vi "S4GUI_003.vi"(7 "Tab ObsEng":enum32{"Obs", "CCD modes", "Guider", "Eng"}(tab)) -> ()   [LabVIEW 2018] (continued)
                    n552 = To Long Integer(number=w1145) -> (32bit integer=w1147:i32)
                    n553 = Subtract(x=w1147, y=w1146) -> (x-y=w1148:i32)
                    n554 = Decrement(x=w1148) -> (x-1=w1150:i32)
                    n555 = Less Than 0?(x=w1150) -> (x < 0?=w1149:bool)
                    n556 = Select(t=0, s=w1149, f=w1150) -> (s? t:f=w1151:i32)
                  }
                }
                "#Pol. Seq. Done" <- w1134
                n557 = Number To Decimal String(number=w1134) -> (decimal integer string=w1135:string)  [unwired: 1 in]
                n558 = Concatenate Strings("#Pol. Seq. Done ", w1135) -> (w1133:string)
                n559 = property on="#Pol. Seq. Done" class="Slide (strict)"("Caption.Text"=w1133) -> ()  [unwired: 2 in, 2 out]
              }
              frame #10 {
                # "OVJ 2022-12-12: \nA visibilidade do Tab ObsEng sempre \nacompanha a habilitação do tab4."
                n560 = Unbundle By Name(w1165) -> ("Cluster ExpMode.tab4"=w1159:T12, "Cluster Polarimetry"=w1186:T23, "Cluster Mode Sync"=w1193:T24)
                n561 = case shown="\"Enabled\", Default" w1159 {
                  tunnel: [TRUE ("Tabs Visible?") w1195] -> w1164
                  frame "Enabled", Default {
                  }
                  frame "Disabled and Grayed Out" {
                    n562 = disable-structure shown="Enabled" {
                      disable-tunnel: [TRUE ("Tabs Visible?") FALSE ("Tabs Visible?")] -> w1195
                      frame Disabled {
                        # "DEBUG"
                      }
                      frame Enabled {
                      }
                    }
                  }
                }
                n563 = property on="Tab Acq Type" class="TabCtl (strict)"("DisabledEnum"=w1159) -> (error out=w1163:errorcluster)  [unwired: 2 in, 1 out]
                n564 = Unbundle By Name(w1193) -> ("Start SM Text"=w1192:string, "Star SM"=w1161:T12, "Pause SM"=w1191:T12, "Stop SM"=w1190:T12, "Abort SM"=w1189:T12, "#Cycles"=w1188:T12, "SSM"=w1187:T12, "Set SM"=w1156:T12, "#Index Cycles"=w1162:T12)
                n565 = property on="Observer" class="Str"(error in=w1163, "DisabledEnum"=w1159) -> (error out=w1158:errorcluster)  [unwired: 1 in, 1 out]
                n566 = property on="Tab ObsEng" class="TabCtl (strict)"("Tabs Visible?"=w1164) -> ()  [unwired: 2 in, 2 out]
                n567 = property on="Project ID" class="Str"(error in=w1158, "DisabledEnum"=w1159) -> (error out=w1157:errorcluster)  [unwired: 1 in, 1 out]
                n568 = property on="set keywords" class="Bool"(error in=w1157, "DisabledEnum"=w1156) -> (error out=w1160:errorcluster)  [unwired: 1 in, 1 out]
                n569 = property on="Start SM" class="Bool"("BoolText.Text"=w1192) -> ()  [unwired: 2 in, 2 out]
                n570 = property on="#Cycles Done" class="Slide (strict)"("DisabledEnum"=w1162) -> ()  [unwired: 2 in, 2 out]
                n571 = property on="Start SM" class="Bool"("DisabledEnum"=w1161) -> ()  [unwired: 2 in, 2 out]
                n572 = property on="Stop SM" class="Bool"("DisabledEnum"=w1190) -> ()  [unwired: 2 in, 2 out]
                n573 = property on="Abort SM" class="Bool"("DisabledEnum"=w1189) -> ()  [unwired: 2 in, 2 out]
                n574 = property on="Pause SM" class="Bool"("DisabledEnum"=w1191) -> ()  [unwired: 2 in, 2 out]
                n575 = property on="# Cycles" class="DigNum (strict)"("DisabledEnum"=w1188) -> ()  [unwired: 2 in, 2 out]
                n576 = property on="SSM" class="Ring (strict)"("DisabledEnum"=w1187) -> ()  [unwired: 2 in, 2 out]
                n577 = property on="set Observer" class="Bool"(error in=w1160, "DisabledEnum"=w1156) -> ()  [unwired: 1 in, 2 out]
                n578 = Unbundle By Name(w1186) -> ("Lambda Selector"=w1185:T12, "Calibrator Selector"=w1184:T12, "Set Waveplate"=w1183:T12, "Select Positions"=w1182:T12, "P0"=w1181:T12, "P8"=w1180:T12, "P1"=w1179:T12, "P9"=w1178:T12, "P2"=w1177:T12, "P10"=w1176:T12, "P3"=w1175:T12, "P11"=w1174:T12, "P4"=w1173:T12, "P12"=w1172:T12, "P5"=w1171:T12, "P13"=w1170:T12, "P6"=w1169:T12, "P14"=w1168:T12, "P7"=w1167:T12, "P15"=w1166:T12)
                n579 = property on="P0" class="Bool (strict)"("DisabledEnum"=w1181) -> ()  [unwired: 2 in, 2 out]
                n580 = property on="Lambda Selector" class="Ring (strict)"("DisabledEnum"=w1185) -> ()  [unwired: 2 in, 2 out]
                n581 = property on="Calibrator Selector" class="Ring (strict)"("DisabledEnum"=w1184) -> ()  [unwired: 2 in, 2 out]
                n582 = property on="Set Waveplate" class="Bool"("DisabledEnum"=w1183) -> ()  [unwired: 2 in, 2 out]
                n583 = property on="P1" class="Bool (strict)"("DisabledEnum"=w1179) -> ()  [unwired: 2 in, 2 out]
                n584 = property on="P2" class="Bool (strict)"("DisabledEnum"=w1177) -> ()  [unwired: 2 in, 2 out]
                n585 = property on="Select Positions" class="Ring (strict)"("DisabledEnum"=w1182) -> ()  [unwired: 2 in, 2 out]
                n586 = property on="P3" class="Bool (strict)"("DisabledEnum"=w1175) -> ()  [unwired: 2 in, 2 out]
                n587 = property on="P4" class="Bool (strict)"("DisabledEnum"=w1173) -> ()  [unwired: 2 in, 2 out]
                n588 = property on="P5" class="Bool (strict)"("DisabledEnum"=w1171) -> ()  [unwired: 2 in, 2 out]
                n589 = property on="P6" class="Bool (strict)"("DisabledEnum"=w1169) -> ()  [unwired: 2 in, 2 out]
                n590 = property on="P7" class="Bool (strict)"("DisabledEnum"=w1167) -> ()  [unwired: 2 in, 2 out]
                n591 = property on="P8" class="Bool (strict)"("DisabledEnum"=w1180) -> ()  [unwired: 2 in, 2 out]
                n592 = property on="P9" class="Bool (strict)"("DisabledEnum"=w1178) -> ()  [unwired: 2 in, 2 out]
                n593 = property on="P10" class="Bool (strict)"("DisabledEnum"=w1176) -> ()  [unwired: 2 in, 2 out]
                n594 = property on="P11" class="Bool (strict)"("DisabledEnum"=w1174) -> ()  [unwired: 2 in, 2 out]
                n595 = property on="P12" class="Bool (strict)"("DisabledEnum"=w1172) -> ()  [unwired: 2 in, 2 out]
                n596 = property on="P15" class="Bool (strict)"("DisabledEnum"=w1166) -> ()  [unwired: 2 in, 2 out]
                n597 = property on="P13" class="Bool (strict)"("DisabledEnum"=w1170) -> ()  [unwired: 2 in, 2 out]
                n598 = property on="P14" class="Bool (strict)"("DisabledEnum"=w1168) -> ()  [unwired: 2 in, 2 out]
              }
              frame #11 {
                n599 = Unbundle By Name(w1212) -> ("Cluster Mode CH1"=w1200:T25, "Cluster Mode Sync"=w1199:T24)
                n600 = Unbundle By Name(w1200) -> ("Start ch1 Text"=w1211:string, "#cycles ch1"=w1210:T12, "Start ch1"=w1209:T12, "Pause ch1"=w1208:T12, "Abort ch1"=w1207:T12, "Stop ch1"=w1206:T12, "Exptime ch1"=w1205:T12, "Exp ch1"=w1204:T12, "Set Cooler"=w1198:T12, "Set Temp"=w1203:T12)
                n601 = Unbundle By Name(w1199) -> ("#Index Cycles"=w1202:T12)
                n602 = case shown="Default" w1202 {
                  tunnel: [T12."Enabled" ("#Index Cycles") T12."Disabled and Grayed Out" ("#Index Cycles")] -> w1201
                  frame "Disabled and Grayed Out" {
                  }
                  frame Default {
                  }
                }
                n603 = property on="Start ch1" class="Bool"("BoolText.Text"=w1211) -> ()  [unwired: 2 in, 2 out]
                n604 = property on="Abort ch1" class="Bool"("DisabledEnum"=w1207) -> ()  [unwired: 2 in, 2 out]
                n605 = property on="Set Temp 1" class="Bool"("DisabledEnum"=w1203) -> ()  [unwired: 2 in, 2 out]
                n606 = property on="Stop ch1" class="Bool"("DisabledEnum"=w1206) -> ()  [unwired: 2 in, 2 out]
                n607 = property on="#cycles ch1" class="DigNum (strict)"("DisabledEnum"=w1210) -> ()  [unwired: 2 in, 2 out]
                n608 = property on="cooler ON 1" class="Bool (strict)"("DisabledEnum"=w1198) -> ()  [unwired: 2 in, 2 out]
                n609 = property on="cooler OFF 1" class="Bool (strict)"("DisabledEnum"=w1198) -> ()  [unwired: 2 in, 2 out]
                n610 = property on="Exptime ch1" class="DigNum (strict)"("DisabledEnum"=w1205) -> ()  [unwired: 2 in, 2 out]
                n611 = property on="Start ch1" class="Bool"("DisabledEnum"=w1209) -> ()  [unwired: 2 in, 2 out]
                n612 = property on="Exp ch1" class="DigNum (strict)"("DisabledEnum"=w1204) -> ()  [unwired: 2 in, 2 out]
                n613 = property on="Cycles Done ch1" class="Slide (strict)"("DisabledEnum"=w1201) -> ()  [unwired: 2 in, 2 out]
                n614 = property on="Pause ch1" class="Bool"("DisabledEnum"=w1208) -> ()  [unwired: 2 in, 2 out]
              }
              frame #12 {
                n615 = Unbundle By Name(w1229) -> ("Cluster Mode CH2"=w1228:T26, "Cluster Mode Sync"=w1217:T24)
                n616 = Unbundle By Name(w1217) -> ("#Index Cycles"=w1218:T12)
                n617 = Unbundle By Name(w1228) -> ("Start ch2 Text"=w1227:string, "#cycles ch2"=w1226:T12, "Start ch2"=w1225:T12, "Pause ch2"=w1224:T12, "Stop ch2"=w1223:T12, "Abort ch2"=w1222:T12, "Exptime ch2"=w1221:T12, "Exp ch2"=w1220:T12, "Set Cooler"=w1215:T12, "Set Temp"=w1219:T12)
                n618 = case shown="\"Disabled and Grayed Out\"" w1218 {
                  tunnel: [T12."Enabled" ("#Index Cycles") T12."Disabled and Grayed Out" ("#Index Cycles")] -> w1216
                  frame "Disabled and Grayed Out" {
                  }
                  frame Default {
                  }
                }
                n619 = property on="Start ch2" class="Bool"("BoolText.Text"=w1227) -> ()  [unwired: 2 in, 2 out]
                n620 = property on="Stop ch2" class="Bool"("DisabledEnum"=w1223) -> ()  [unwired: 2 in, 2 out]
                n621 = property on="Abort ch2" class="Bool"("DisabledEnum"=w1222) -> ()  [unwired: 2 in, 2 out]
                n622 = property on="#cycles ch2" class="DigNum (strict)"("DisabledEnum"=w1226) -> ()  [unwired: 2 in, 2 out]
                n623 = property on="Set Temp 2" class="Bool"("DisabledEnum"=w1219) -> ()  [unwired: 2 in, 2 out]
                n624 = property on="Exptime ch2" class="DigNum (strict)"("DisabledEnum"=w1221) -> ()  [unwired: 2 in, 2 out]
                n625 = property on="cooler OFF 2" class="Bool (strict)"("DisabledEnum"=w1215) -> ()  [unwired: 2 in, 2 out]
                n626 = property on="cooler ON 2" class="Bool (strict)"("DisabledEnum"=w1215) -> ()  [unwired: 2 in, 2 out]
                n627 = property on="Start ch2" class="Bool"("DisabledEnum"=w1225) -> ()  [unwired: 2 in, 2 out]
                n628 = property on="Cycles Done ch2" class="Slide (strict)"("DisabledEnum"=w1216) -> ()  [unwired: 2 in, 2 out]
                n629 = property on="Exp ch2" class="DigNum (strict)"("DisabledEnum"=w1220) -> ()  [unwired: 2 in, 2 out]
                n630 = property on="Pause ch2" class="Bool"("DisabledEnum"=w1224) -> ()  [unwired: 2 in, 2 out]
              }
              frame #13 {
                n631 = Unbundle By Name(w1246) -> ("Cluster Mode CH3"=w1245:T27, "Cluster Mode Sync"=w1234:T24)
                n632 = Unbundle By Name(w1234) -> ("#Index Cycles"=w1235:T12)
                n633 = Unbundle By Name(w1245) -> ("Start ch3 Text"=w1244:string, "#cycles ch3"=w1243:T12, "Start ch3"=w1242:T12, "Pause ch3"=w1241:T12, "Stop ch3"=w1240:T12, "Abort ch3"=w1239:T12, "Exptime ch3"=w1238:T12, "Exp ch3"=w1237:T12, "Set Cooler"=w1232:T12, "Set Temp"=w1236:T12)
                n634 = case shown="\"Disabled and Grayed Out\"" w1235 {
                  tunnel: [T12."Enabled" ("#Index Cycles") T12."Disabled and Grayed Out" ("#Index Cycles")] -> w1233
                  frame "Disabled and Grayed Out" {
                  }
                  frame Default {
                  }
                }
                n635 = property on="Start ch3" class="Bool"("BoolText.Text"=w1244) -> ()  [unwired: 2 in, 2 out]
                n636 = property on="Stop ch3" class="Bool"("DisabledEnum"=w1240) -> ()  [unwired: 2 in, 2 out]
                n637 = property on="Abort ch3" class="Bool"("DisabledEnum"=w1239) -> ()  [unwired: 2 in, 2 out]
                n638 = property on="Cycles Done ch3" class="Slide (strict)"("DisabledEnum"=w1233) -> ()  [unwired: 2 in, 2 out]
                n639 = property on="#cycles ch3" class="DigNum (strict)"("DisabledEnum"=w1243) -> ()  [unwired: 2 in, 2 out]
                n640 = property on="cooler OFF 3" class="Bool (strict)"("DisabledEnum"=w1232) -> ()  [unwired: 2 in, 2 out]
                n641 = property on="Set Temp 3" class="Bool"("DisabledEnum"=w1236) -> ()  [unwired: 2 in, 2 out]
                n642 = property on="cooler ON 3" class="Bool (strict)"("DisabledEnum"=w1232) -> ()  [unwired: 2 in, 2 out]
                n643 = property on="Exptime ch3" class="DigNum (strict)"("DisabledEnum"=w1238) -> ()  [unwired: 2 in, 2 out]
                n644 = property on="Start ch3" class="Bool"("DisabledEnum"=w1242) -> ()  [unwired: 2 in, 2 out]
                n645 = property on="Exp ch3" class="DigNum (strict)"("DisabledEnum"=w1237) -> ()  [unwired: 2 in, 2 out]
                n646 = property on="Pause ch3" class="Bool"("DisabledEnum"=w1241) -> ()  [unwired: 2 in, 2 out]
              }
              frame #14 {
                n647 = Unbundle By Name(w1263) -> ("Cluster Mode CH4"=w1262:T28, "Cluster Mode Sync"=w1251:T24)
                n648 = Unbundle By Name(w1251) -> ("#Index Cycles"=w1252:T12)
                n649 = Unbundle By Name(w1262) -> ("Start ch4 Text"=w1261:string, "#cycles ch4"=w1260:T12, "Start ch4"=w1259:T12, "Pause ch4"=w1258:T12, "Stop ch4"=w1257:T12, "Abort ch4"=w1256:T12, "Exptime ch4"=w1255:T12, "Exp ch4"=w1254:T12, "Set Cooler"=w1249:T12, "Set Temp"=w1253:T12)
                n650 = case shown="\"Disabled and Grayed Out\"" w1252 {
                  tunnel: [T12."Enabled" ("#Index Cycles") T12."Disabled and Grayed Out" ("#Index Cycles")] -> w1250
                  frame "Disabled and Grayed Out" {
                  }
                  frame Default {
                  }
                }
                n651 = property on="Start ch4" class="Bool"("BoolText.Text"=w1261) -> ()  [unwired: 2 in, 2 out]
                n652 = property on="Stop ch4" class="Bool"("DisabledEnum"=w1257) -> ()  [unwired: 2 in, 2 out]
                n653 = property on="Abort ch4" class="Bool"("DisabledEnum"=w1256) -> ()  [unwired: 2 in, 2 out]
                n654 = property on="#cycles ch4" class="DigNum (strict)"("DisabledEnum"=w1260) -> ()  [unwired: 2 in, 2 out]
                n655 = property on="Set Temp 4" class="Bool"("DisabledEnum"=w1253) -> ()  [unwired: 2 in, 2 out]
                n656 = property on="cooler ON 4" class="Bool (strict)"("DisabledEnum"=w1249) -> ()  [unwired: 2 in, 2 out]
                n657 = property on="cooler OFF 4" class="Bool (strict)"("DisabledEnum"=w1249) -> ()  [unwired: 2 in, 2 out]
                n658 = property on="Exptime ch4" class="DigNum (strict)"("DisabledEnum"=w1255) -> ()  [unwired: 2 in, 2 out]
                n659 = property on="Cycles Done ch4" class="Slide (strict)"("DisabledEnum"=w1250) -> ()  [unwired: 2 in, 2 out]
                n660 = property on="Start ch4" class="Bool"("DisabledEnum"=w1259) -> ()  [unwired: 2 in, 2 out]
                n661 = property on="Exp ch4" class="DigNum (strict)"("DisabledEnum"=w1254) -> ()  [unwired: 2 in, 2 out]
                n662 = property on="Pause ch4" class="Bool"("DisabledEnum"=w1258) -> ()  [unwired: 2 in, 2 out]
              }
              frame #15 {
                # "Carrega coluna do Channel 1"
                # "Aba:  Eng->Camera"
                n663 = Unbundle By Name(w1330) -> ("ChannelA_CCD"=w1275:T29, "CHA_Checked Params"=w1321:T14, "ChannelA_Status.connection"=w1274:bool)
                n664 = Unbundle By Name(w1321) -> ("ACQUISITION_MODE"=w1299:bool, "TRIGGER_MODE"=w1300:bool, "READ_MODE"=w1301:bool, "PREAMP"=w1309:bool, "READOUT_RATE"=w1310:bool, "VERTICAL_SHIFT_SPEED"=w1311:bool, "EM_MODE"=w1312:bool, "EM_GAIN"=w1302:bool, "SHUTTER_MODE"=w1303:bool, "SHUTTER_TTL"=w1304:bool, "SHUTTER_OPENING_TIME"=w1305:bool, "SHUTTER_CLOSING_TIME"=w1306:bool, "VBIN"=w1307:bool, "HBIN"=w1308:bool, "INITIAL_LINE"=w1313:bool, "INITIAL_COLUMN"=w1318:bool, "FINAL_LINE"=w1320:bool, "FINAL_COLUMN"=w1317:bool, "FRAME_TRANSFER"=w1316:bool, "VERTICAL_CLOCK_VOLTAGE"=w1315:bool, "AD_CHANNEL"=w1314:bool)
                n665 = local read "CH1on"() -> (w1267:bool)
                n666 = Unbundle By Name(w1275) -> ("INITIAL_LINE"=w1297:u16, "INITIAL_COLUMN"=w1296:u16, "FINAL_LINE"=w1295:u16, "FINAL_COLUMN"=w1294:u16, "VBIN"=w1293:u16, "HBIN"=w1292:u16, "PREAMP"=w1291:u8, "EM_GAIN"=w1290:u16, "READOUT_RATE"=w1289:u8, "SHUTTER_OPENNING_TIME"=w1288:u16, "SHUTTER_CLOSING_TIME"=w1287:u16, "VERTICAL_SHIFT_SPEED"=w1286:u8, "READ_MODE"=w1285:u8, "VERTICAL_CLOCK_VOLTAGE"=w1284:u8, "AD_CHANNEL"=w1283:u32, "SHUTTER_MODE"=w1282:u8, "SHUTTER_TTL"=w1281:u8, "TRIGGER_MODE"=w1280:u8, "FRAME_TRANSFER"=w1279:bool, "ACQUISITION_MODE"=w1277:u8, "EM_MODE"=w1276:u8)
                n667 = Equal?(x=w1325, y="none") -> (x = y?=w1322:bool)
                n668 = Equal?(x=w1325, y="default.cfg") -> (x = y?=w1323:bool)
                n669 = Or(x=w1323, y=w1322) -> (x .or. y?=w1324:bool)
                n670 = case shown="True" w1324 {
                  tunnel: [T12."Enabled" ("Disabled") T12."Disabled and Grayed Out" ("Disabled")] -> w1327
                  frame False {
                    # "Se Curr Conf File != default.cfg,\nhabilita botão de Salvar."
                  }
                  frame True {
                    # "Não é permitido salvar em \ncima de default.cfg"
                  }
                }
                n671 = case shown="True" w1274 {
                  tunnel: w1275 -> [_ w1383]
                  tunnel: [w1376 w1382] -> w1273
                  tunnel: [w1376 w1381] -> w1272
                  tunnel: [w1376 w1380] -> w1271
                  tunnel: [w1376 w1379] -> w1270
                  tunnel: [w1376 w1378] -> w1269
                  tunnel: [w1376 w1377] -> w1268
                  frame False {
                    w1376 = "" ("RO1")
                  }
                  frame True {
                    n672 = stacked-sequence "Atualizacao dos indicadores inferiores do CANAL A da tela principal" {
                      tunnel: w1383 -> [w1398 w1401 w1406 w1415 w1418 w1422]
                      tunnel: [w1384 _ _ _ _ _] -> w1382
                      tunnel: [_ w1399 _ _ _ _] -> w1381
                      tunnel: [_ _ w1404 _ _ _] -> w1380
                      tunnel: [_ _ _ w1409 _ _] -> w1379
                      tunnel: [_ _ _ _ w1416 _] -> w1378
                      tunnel: [_ _ _ _ _ w1419] -> w1377
                      frame #0 {
                        # "SubImage"
                        n673 = Unbundle By Name(w1398) -> ("INITIAL_LINE"=w1396:u16, "FINAL_LINE"=w1395:u16, "INITIAL_COLUMN"=w1394:u16, "FINAL_COLUMN"=w1393:u16)
                        n674 = Number To Decimal String(number=w1396) -> (decimal integer string=w1392:string)  [unwired: 1 in]
                        n675 = Number To Decimal String(number=w1395) -> (decimal integer string=w1390:string)  [unwired: 1 in]
                        n676 = Number To Decimal String(number=w1394) -> (decimal integer string=w1388:string)  [unwired: 1 in]
                        n677 = Number To Decimal String(number=w1393) -> (decimal integer string=w1386:string)  [unwired: 1 in]
                        n678 = Concatenate Strings("[", w1392, ":", w1390, ",", w1388, ":", w1386, "]") -> (w1384:string)
                      }
                      frame #1 {
                        # "Em Active"
                        n679 = Unbundle By Name(w1401) -> ("EM_MODE"=w1400:u8)
                        n680 = case shown="0, Default" w1400 {
                          tunnel: ["Electron M." ("EmActive1") "Convent." ("EmActive1")] -> w1399
                          frame 0, Default {
                          }
                          frame 1 {
                          }
                        }
                      }
                      frame #2 {
                        # "Pre Amp"
                        n681 = Unbundle By Name(w1406) -> ("PREAMP"=w1405:u8)
                        n682 = case shown="1" w1405 {
                          tunnel: ["Gain 1" ("EmActive1") "Gain 2" ("EmActive1")] -> w1404
                          frame 0, Default {
                          }
                          frame 1 {
                          }
                        }
                      }
                      frame #3 {
                        # "Binning"
                        n683 = Unbundle By Name(w1415) -> ("VBIN"=w1414:u16, "HBIN"=w1413:u16)
                        n684 = Number To Decimal String(number=w1413) -> (decimal integer string=w1410:string)  [unwired: 1 in]
                        n685 = Number To Decimal String(number=w1414) -> (decimal integer string=w1412:string)  [unwired: 1 in]
                        n686 = Concatenate Strings(w1412, "x", w1410) -> (w1409:string)
                      }
                      frame #4 {
                        # "Gain"
                        n687 = Unbundle By Name(w1418) -> ("EM_GAIN"=w1417:u16)
                        n688 = Number To Decimal String(number=w1417) -> (decimal integer string=w1416:string)  [unwired: 1 in]
                      }
                      frame #5 {
                        # "Readout"
                        n689 = Unbundle By Name(w1422) -> ("EM_MODE"=w1421:u8, "READOUT_RATE"=w1420:u8)
                        n690 = case shown="0, Default" w1421 {
                          tunnel: w1420 -> [w1424 w1430]
                          tunnel: [w1423 w1429] -> w1419
                          frame 0, Default {
                            n691 = case shown="0, Default" w1424 {
                              tunnel: ["30 MHz" ("EmActive1") "20 MHz" ("EmActive1") "10 MHz" ("EmActive1") "1 MHz" ("EmActive1")] -> w1423
                              frame 0, Default {
                              }
                              frame 1 {
                              }
                              frame 2 {
                              }
                              frame 3 {
                              }
                            }
                          }
                          frame 1 {
                            n692 = case shown="1" w1430 {
                              tunnel: ["1 MHz" ("EmActive1") "0.1 MHz" ("EmActive1")] -> w1429
                              frame 0, Default {
                              }
                              frame 1 {
                              }
                            }
                          }
                        }
                      }
                    }
                  }
                }
                n693 = case shown="False" w1267 {
                  tunnel: w1320 -> [_ w1375]
                  tunnel: w1318 -> [_ w1371]
                  tunnel: w1317 -> [_ w1369]
                  tunnel: w1316 -> [_ w1365]
                  tunnel: w1315 -> [_ w1364]
                  tunnel: w1314 -> [_ w1363]
                  tunnel: w1313 -> [_ w1355]
                  tunnel: w1312 -> [_ w1347]
                  tunnel: w1311 -> [_ w1346]
                  tunnel: w1310 -> [_ w1345]
                  tunnel: w1309 -> [_ w1344]
                  tunnel: w1308 -> [_ w1343]
                  tunnel: w1307 -> [_ w1342]
                  tunnel: w1306 -> [_ w1341]
                  tunnel: w1305 -> [_ w1340]
                  tunnel: w1304 -> [_ w1339]
                  tunnel: w1303 -> [_ w1338]
                  tunnel: w1302 -> [_ w1337]
                  tunnel: w1301 -> [_ w1336]
                  tunnel: w1300 -> [_ w1335]
                  tunnel: w1299 -> [_ w1334]
                  tunnel: [T12."Disabled and Grayed Out" ("Disabled") T12."Enabled" ("Disabled")] -> w1266
                  frame False {
                    w1331 = FALSE
                    n694 = property on="Image FInal Column" class="DigNum (strict)"("Blinking"=w1331) -> ()  [unwired: 2 in, 2 out]
                    n695 = property on="Frame Transfer" class="Bool (strict)"("Blinking"=w1331) -> ()  [unwired: 2 in, 2 out]
                    n696 = property on="Vertical Clock Voltage" class="Ring (strict)"("Blinking"=w1331) -> ()  [unwired: 2 in, 2 out]
                    n697 = property on="A/D  Channel" class="DigNum (strict)"("Blinking"=w1331) -> ()  [unwired: 2 in, 2 out]
                    n698 = property on="Image Initial Line" class="DigNum (strict)"("Blinking"=w1331) -> ()  [unwired: 2 in, 2 out]
                    n699 = property on="Image Initial Column" class="DigNum (strict)"("Blinking"=w1331) -> ()  [unwired: 2 in, 2 out]
                    n700 = property on="Image Final Line" class="DigNum (strict)"("Blinking"=w1331) -> ()  [unwired: 2 in, 2 out]
                    n701 = property on="Shutter Openning Time" class="DigNum (strict)"("Blinking"=w1331) -> ()  [unwired: 2 in, 2 out]
                    n702 = property on="Shutter Closing Time" class="DigNum (strict)"("Blinking"=w1331) -> ()  [unwired: 2 in, 2 out]
                    n703 = property on="Vertical Binning" class="DigNum (strict)"("Blinking"=w1331) -> ()  [unwired: 2 in, 2 out]
                    n704 = property on="Horizontal Binning" class="DigNum (strict)"("Blinking"=w1331) -> ()  [unwired: 2 in, 2 out]
                    n705 = property on="CCD EM Gain" class="DigNum (strict)"("Blinking"=w1331) -> ()  [unwired: 2 in, 2 out]
                    n706 = property on="Shutter Mode" class="Ring (strict)"("Blinking"=w1331) -> ()  [unwired: 2 in, 2 out]
                    n707 = property on="Shutter TTL" class="Ring (strict)"("Blinking"=w1331) -> ()  [unwired: 2 in, 2 out]
                    n708 = property on="Acquisition Mode" class="Ring (strict)"("Blinking"=w1331) -> ()  [unwired: 2 in, 2 out]
                    n709 = property on="Readout Rate" class="Ring (strict)"("Blinking"=w1331) -> ()  [unwired: 2 in, 2 out]
                    n710 = property on="Vertical Shift Speed" class="Ring (strict)"("Blinking"=w1331) -> ()  [unwired: 2 in, 2 out]
                    n711 = property on="CCD EM Mode" class="Ring (strict)"("Blinking"=w1331) -> ()  [unwired: 2 in, 2 out]
                    n712 = property on="Trigger Mode" class="Ring (strict)"("Blinking"=w1331) -> ()  [unwired: 2 in, 2 out]
                    n713 = property on="Read Mode" class="Ring (strict)"("Blinking"=w1331) -> ()  [unwired: 2 in, 2 out]
                    n714 = property on="Pre-amplification Gain" class="Ring (strict)"("Blinking"=w1331) -> ()  [unwired: 2 in, 2 out]
                  }
                  frame True {
                    n715 = Not(x=w1369) -> (.not. x?=w1370:bool)
                    n716 = Not(x=w1365) -> (.not. x?=w1367:bool)
                    n717 = Not(x=w1364) -> (.not. x?=w1368:bool)
                    n718 = Not(x=w1363) -> (.not. x?=w1366:bool)
                    n719 = Not(x=w1355) -> (.not. x?=w1373:bool)
                    n720 = Not(x=w1371) -> (.not. x?=w1372:bool)
                    n721 = Not(x=w1375) -> (.not. x?=w1374:bool)
                    n722 = property on="Image FInal Column" class="DigNum (strict)"("Blinking"=w1370) -> ()  [unwired: 2 in, 2 out]
                    n723 = property on="Frame Transfer" class="Bool (strict)"("Blinking"=w1367) -> ()  [unwired: 2 in, 2 out]
                    n724 = property on="Vertical Clock Voltage" class="Ring (strict)"("Blinking"=w1368) -> ()  [unwired: 2 in, 2 out]
                    n725 = property on="A/D  Channel" class="DigNum (strict)"("Blinking"=w1366) -> ()  [unwired: 2 in, 2 out]
                    n726 = property on="Image Initial Line" class="DigNum (strict)"("Blinking"=w1373) -> ()  [unwired: 2 in, 2 out]
                    n727 = property on="Image Initial Column" class="DigNum (strict)"("Blinking"=w1372) -> ()  [unwired: 2 in, 2 out]
                    n728 = property on="Image Final Line" class="DigNum (strict)"("Blinking"=w1374) -> ()  [unwired: 2 in, 2 out]
                    n729 = Not(x=w1340) -> (.not. x?=w1359:bool)
                    n730 = Not(x=w1341) -> (.not. x?=w1361:bool)
                    n731 = Not(x=w1342) -> (.not. x?=w1360:bool)
                    n732 = Not(x=w1343) -> (.not. x?=w1362:bool)
                    n733 = Not(x=w1337) -> (.not. x?=w1357:bool)
                    n734 = Not(x=w1338) -> (.not. x?=w1358:bool)
                    n735 = Not(x=w1339) -> (.not. x?=w1356:bool)
                    n736 = property on="Shutter Openning Time" class="DigNum (strict)"("Blinking"=w1359) -> ()  [unwired: 2 in, 2 out]
                    n737 = property on="Shutter Closing Time" class="DigNum (strict)"("Blinking"=w1361) -> ()  [unwired: 2 in, 2 out]
                    n738 = property on="Vertical Binning" class="DigNum (strict)"("Blinking"=w1360) -> ()  [unwired: 2 in, 2 out]
                    n739 = property on="Horizontal Binning" class="DigNum (strict)"("Blinking"=w1362) -> ()  [unwired: 2 in, 2 out]
                    n740 = property on="CCD EM Gain" class="DigNum (strict)"("Blinking"=w1357) -> ()  [unwired: 2 in, 2 out]
                    n741 = property on="Shutter Mode" class="Ring (strict)"("Blinking"=w1358) -> ()  [unwired: 2 in, 2 out]
                    n742 = property on="Shutter TTL" class="Ring (strict)"("Blinking"=w1356) -> ()  [unwired: 2 in, 2 out]
                    n743 = Not(x=w1334) -> (.not. x?=w1348:bool)
                    n744 = Not(x=w1345) -> (.not. x?=w1351:bool)
                    n745 = Not(x=w1346) -> (.not. x?=w1349:bool)
                    n746 = Not(x=w1347) -> (.not. x?=w1350:bool)
                    n747 = Not(x=w1335) -> (.not. x?=w1353:bool)
                    n748 = Not(x=w1336) -> (.not. x?=w1352:bool)
                    n749 = Not(x=w1344) -> (.not. x?=w1354:bool)
                    n750 = property on="Acquisition Mode" class="Ring (strict)"("Blinking"=w1348) -> ()  [unwired: 2 in, 2 out]
                    n751 = property on="Readout Rate" class="Ring (strict)"("Blinking"=w1351) -> ()  [unwired: 2 in, 2 out]
                    n752 = property on="Vertical Shift Speed" class="Ring (strict)"("Blinking"=w1349) -> ()  [unwired: 2 in, 2 out]
                    n753 = property on="CCD EM Mode" class="Ring (strict)"("Blinking"=w1350) -> ()  [unwired: 2 in, 2 out]
                    n754 = property on="Trigger Mode" class="Ring (strict)"("Blinking"=w1353) -> ()  [unwired: 2 in, 2 out]
                    n755 = property on="Read Mode" class="Ring (strict)"("Blinking"=w1352) -> ()  [unwired: 2 in, 2 out]
                    n756 = property on="Pre-amplification Gain" class="Ring (strict)"("Blinking"=w1354) -> ()  [unwired: 2 in, 2 out]
                  }
                }
                n757 = property on="Save Button" class="Bool (strict)"("DisabledEnum"=w1327) -> ()  [unwired: 2 in, 2 out]
                n758 = First Call?() -> (First Call?: T/F=w1298:bool)
                n759 = case shown="True" w1298 {
                  tunnel: w1297 -> [_ w1453]
                  tunnel: w1296 -> [_ w1452]
                  tunnel: w1295 -> [_ w1451]
                  tunnel: w1294 -> [_ w1450]
                  tunnel: w1293 -> [_ w1449]
                  tunnel: w1292 -> [_ w1448]
                  tunnel: w1291 -> [_ w1447]
                  tunnel: w1290 -> [_ w1446]
                  tunnel: w1289 -> [_ w1445]
                  tunnel: w1288 -> [_ w1444]
                  tunnel: w1287 -> [_ w1443]
                  tunnel: w1286 -> [_ w1442]
                  tunnel: w1285 -> [_ w1441]
                  tunnel: w1284 -> [_ w1440]
                  tunnel: w1283 -> [_ w1439]
                  tunnel: w1282 -> [_ w1438]
                  tunnel: w1281 -> [_ w1437]
                  tunnel: w1280 -> [_ w1436]
                  tunnel: w1279 -> [_ w1435]
                  tunnel: w1277 -> [_ w1434]
                  tunnel: w1276 -> [_ w1433]
                  frame False {
                  }
                  frame True {
                    n760 = local read "Input Cluster"() -> (w1457:T8)
                    n761 = Unbundle By Name(w1457) -> ("Parameters"=w1455:T5)
                    n762 = Bundle By Name(cluster=w1455, "Image \nInitial Line"=w1453, "Image\nInitial Column"=w1452, "Image\nFinal Line"=w1451, "Image\nFInal Column"=w1450, "Vertical\nBinning"=w1449, "Horizontal\nBinning"=w1448, "Pre-amplification\nGain"=w1447, "CCD\nEM Gain"=w1446, "Readout\nRate"=w1445, "Shutter\nOpenning Time"=w1444, "Shutter\nClosing Time"=w1443, "Vertical\nShift Speed"=w1442, "Read\nMode"=w1441, "Vertical\nClock Voltage"=w1440, "A/D \nChannel"=w1439, "Shutter\nMode"=w1438, "Shutter\nTTL"=w1437, "Trigger\nMode"=w1436, "Frame\nTransfer"=w1435, "Acquisition\nMode"=w1434, "CCD \nEM Mode"=w1433) -> (w1454:T5)
                    n763 = Bundle By Name(cluster=w1457, "Parameters"=w1454) -> (w1456:T8)
                    n764 = local write "Input Cluster"(w1456) -> ()
                  }
                }
                n765 = local read "Cameras Cluster"() -> (w1329:T7)
                n766 = Bundle By Name(cluster=w1329, "Current Configuration.Image Initial Line"=w1297, "Current Configuration.Image Initial Column"=w1296, "Current Configuration.Image Final Line"=w1295, "Current Configuration.Image FInal Column"=w1294, "Current Configuration.Vertical Binning"=w1293, "Current Configuration.Horizontal Binning"=w1292, "Current Configuration.Pre-amplification Gain"=w1291, "Current Configuration.CCD EM Gain"=w1290, "Current Configuration.Readout Rate"=w1289, "Current Configuration.Shutter Openning Time"=w1288, "Current Configuration.Shutter Closing Time"=w1287, "Current Configuration.Vertical Shift Speed"=w1286, "Current Configuration.Read Mode"=w1285, "Current Configuration.Vertical Clock Voltage"=w1284, "Current Configuration.A/D  Channel"=w1283, "Current Configuration.Shutter Mode"=w1282, "Current Configuration.Shutter TTL"=w1281, "Current Configuration.Trigger Mode"=w1280, "Current Configuration.Frame Transfer"=w1279, "Current Configuration.Acquisition Mode"=w1277, "Current Configuration.CCD EM Mode"=w1276) -> (w1278:T7)
                n767 = local write "RO1"(w1268) -> ()
                n768 = local write "SI1"(w1273) -> ()
                n769 = local write "EA1"(w1272) -> ()
                n770 = local write "PA1"(w1271) -> ()
                n771 = local write "B1"(w1270) -> ()
                n772 = local write "G1"(w1269) -> ()
                n773 = local write "Cameras Cluster"(w1278) -> ()
                n774 = Compound Arithmetic op=AND(w1299, w1300, w1301, w1309, w1310, w1311, w1312, w1302, w1303, w1304, w1305, w1306, w1307, w1308, w1313, w1318, w1320, w1317, w1316, w1315, w1314) -> (→"CCD checked 1":bool)
                n775 = property on="Shutter Openning Time" class="DigNum (strict)"("DisabledEnum"=w1266) -> ()  [unwired: 2 in, 2 out]
                n776 = property on="Shutter Closing Time" class="DigNum (strict)"("DisabledEnum"=w1266) -> ()  [unwired: 2 in, 2 out]
                n777 = property on="Vertical Binning" class="DigNum (strict)"("DisabledEnum"=w1266) -> ()  [unwired: 2 in, 2 out]
                n778 = property on="Horizontal Binning" class="DigNum (strict)"("DisabledEnum"=w1266) -> ()  [unwired: 2 in, 2 out]
                n779 = property on="CCD EM Gain" class="DigNum (strict)"("DisabledEnum"=w1266) -> ()  [unwired: 2 in, 2 out]
                n780 = property on="Shutter Mode" class="Ring (strict)"("DisabledEnum"=w1266) -> ()  [unwired: 2 in, 2 out]
                n781 = property on="Shutter TTL" class="Ring (strict)"("DisabledEnum"=w1266) -> ()  [unwired: 2 in, 2 out]
                n782 = property on="Acquisition Mode" class="Ring (strict)"("DisabledEnum"=w1266) -> ()  [unwired: 2 in, 2 out]
                n783 = property on="Readout Rate" class="Ring (strict)"("DisabledEnum"=w1266) -> ()  [unwired: 2 in, 2 out]
                n784 = property on="Vertical Shift Speed" class="Ring (strict)"("DisabledEnum"=w1266) -> ()  [unwired: 2 in, 2 out]
                n785 = property on="CCD EM Mode" class="Ring (strict)"("DisabledEnum"=w1266) -> ()  [unwired: 2 in, 2 out]
                n786 = property on="Trigger Mode" class="Ring (strict)"("DisabledEnum"=w1266) -> ()  [unwired: 2 in, 2 out]
                n787 = property on="Read Mode" class="Ring (strict)"("DisabledEnum"=w1266) -> ()  [unwired: 2 in, 2 out]
                n788 = property on="Pre-amplification Gain" class="Ring (strict)"("DisabledEnum"=w1266) -> ()  [unwired: 2 in, 2 out]
                n789 = property on="Image FInal Column" class="DigNum (strict)"("DisabledEnum"=w1266) -> ()  [unwired: 2 in, 2 out]
                n790 = property on="Frame Transfer" class="Bool (strict)"("DisabledEnum"=w1266) -> ()  [unwired: 2 in, 2 out]
                n791 = property on="Vertical Clock Voltage" class="Ring (strict)"("DisabledEnum"=w1266) -> ()  [unwired: 2 in, 2 out]
                n792 = property on="A/D  Channel" class="DigNum (strict)"("DisabledEnum"=w1266) -> ()  [unwired: 2 in, 2 out]
                n793 = property on="Image Initial Line" class="DigNum (strict)"("DisabledEnum"=w1266) -> ()  [unwired: 2 in, 2 out]
                n794 = property on="Image Initial Column" class="DigNum (strict)"("DisabledEnum"=w1266) -> ()  [unwired: 2 in, 2 out]
                n795 = property on="Image Final Line" class="DigNum (strict)"("DisabledEnum"=w1266) -> ()  [unwired: 2 in, 2 out]
                "Current Configuration File:" <- w1325
              }
              frame #16 {
                # "Carrega coluna do Channel 2"
                # "Aba:  Eng->Camera"
                n796 = Unbundle By Name(w1516) -> ("ChannelB_CCD"=w1472:T29, "CHB_Checked Params"=w1473:T14, "ChannelB_Status.connection"=w1471:bool)
                n797 = Unbundle By Name(w1473) -> ("ACQUISITION_MODE"=w1489:bool, "TRIGGER_MODE"=w1488:bool, "READ_MODE"=w1487:bool, "PREAMP"=w1486:bool, "READOUT_RATE"=w1462:bool, "VERTICAL_SHIFT_SPEED"=w1461:bool, "EM_MODE"=w1485:bool, "EM_GAIN"=w1496:bool, "SHUTTER_MODE"=w1495:bool, "SHUTTER_TTL"=w1494:bool, "SHUTTER_OPENING_TIME"=w1493:bool, "SHUTTER_CLOSING_TIME"=w1492:bool, "VBIN"=w1491:bool, "HBIN"=w1490:bool, "INITIAL_LINE"=w1503:bool, "INITIAL_COLUMN"=w1502:bool, "FINAL_LINE"=w1501:bool, "FINAL_COLUMN"=w1500:bool, "FRAME_TRANSFER"=w1499:bool, "VERTICAL_CLOCK_VOLTAGE"=w1498:bool, "AD_CHANNEL"=w1497:bool)
                n798 = case shown="True" w1471 {
                  tunnel: w1472 -> [_ w1573]
                  tunnel: [w1566 w1572] -> w1470
                  tunnel: [w1566 w1571] -> w1469
                  tunnel: [w1566 w1570] -> w1468
                  tunnel: [w1566 w1569] -> w1467
                  tunnel: [w1566 w1568] -> w1466
                  tunnel: [w1566 w1567] -> w1465
                  frame False {
                    w1566 = "" ("EmActive1")
                  }
                  frame True {
                    n799 = stacked-sequence "Atualizacao dos indicadores inferiores do CANAL B da tela principal" {
                      tunnel: w1573 -> [w1588 w1591 w1596 w1605 w1608 w1612]
                      tunnel: [_ w1589 _ _ _ _] -> w1572
                      tunnel: [_ _ w1594 _ _ _] -> w1571
                      tunnel: [_ _ _ w1599 _ _] -> w1570
                      tunnel: [_ _ _ _ w1606 _] -> w1569
                      tunnel: [_ _ _ _ _ w1609] -> w1568
                      tunnel: [w1574 _ _ _ _ _] -> w1567
                      frame #0 {
                        # "SubImage"
                        n800 = Unbundle By Name(w1588) -> ("INITIAL_LINE"=w1586:u16, "FINAL_LINE"=w1585:u16, "INITIAL_COLUMN"=w1584:u16, "FINAL_COLUMN"=w1583:u16)
                        n801 = Number To Decimal String(number=w1586) -> (decimal integer string=w1582:string)  [unwired: 1 in]
                        n802 = Number To Decimal String(number=w1585) -> (decimal integer string=w1580:string)  [unwired: 1 in]
                        n803 = Number To Decimal String(number=w1584) -> (decimal integer string=w1578:string)  [unwired: 1 in]
                        n804 = Number To Decimal String(number=w1583) -> (decimal integer string=w1576:string)  [unwired: 1 in]
                        n805 = Concatenate Strings("[", w1582, ":", w1580, ",", w1578, ":", w1576, "]") -> (w1574:string)
                      }
                      frame #1 {
                        # "Em Active"
                        n806 = Unbundle By Name(w1591) -> ("EM_MODE"=w1590:u8)
                        n807 = case shown="0, Default" w1590 {
                          tunnel: ["Electron M." ("EmActive1") "Convent." ("EmActive1")] -> w1589
                          frame 0, Default {
                          }
                          frame 1 {
                          }
                        }
                      }
                      frame #2 {
                        # "Pre Amp"
                        n808 = Unbundle By Name(w1596) -> ("PREAMP"=w1595:u8)
                        n809 = case shown="1" w1595 {
                          tunnel: ["Gain 1" ("EmActive1") "Gain 2" ("EmActive1")] -> w1594
                          frame 0, Default {
                          }
                          frame 1 {
                          }
                        }
                      }
                      frame #3 {
                        # "Binning"
                        n810 = Unbundle By Name(w1605) -> ("VBIN"=w1604:u16, "HBIN"=w1603:u16)
                        n811 = Number To Decimal String(number=w1603) -> (decimal integer string=w1601:string)  [unwired: 1 in]
                        n812 = Number To Decimal String(number=w1604) -> (decimal integer string=w1602:string)  [unwired: 1 in]
                        n813 = Concatenate Strings(w1602, "x", w1601) -> (w1599:string)
                      }
                      frame #4 {
                        # "Gain"
                        n814 = Unbundle By Name(w1608) -> ("EM_GAIN"=w1607:u16)
                        n815 = Number To Decimal String(number=w1607) -> (decimal integer string=w1606:string)  [unwired: 1 in]
                      }
                      frame #5 {
                        # "Readout"
                        n816 = Unbundle By Name(w1612) -> ("EM_MODE"=w1611:u8, "READOUT_RATE"=w1610:u8)
                        n817 = case shown="0, Default" w1611 {
                          tunnel: w1610 -> [w1614 w1620]
                          tunnel: [w1613 w1619] -> w1609
                          frame 0, Default {
                            n818 = case shown="3" w1614 {
                              tunnel: ["30 MHz" ("EmActive1") "20 MHz" ("EmActive1") "10 MHz" ("EmActive1") "1 MHz" ("EmActive1")] -> w1613
                              frame 0, Default {
                              }
                              frame 1 {
                              }
                              frame 2 {
                              }
                              frame 3 {
                              }
                            }
                          }
                          frame 1 {
                            n819 = case shown="1" w1620 {
                              tunnel: ["1 MHz" ("EmActive1") "0.1 MHz" ("EmActive1")] -> w1619
                              frame 0, Default {
                              }
                              frame 1 {
                              }
                            }
                          }
                        }
                      }
                    }
                  }
                }
                n820 = Unbundle By Name(w1472) -> ("INITIAL_LINE"=w1478:u16, "INITIAL_COLUMN"=w1476:u16, "FINAL_LINE"=w1479:u16, "FINAL_COLUMN"=w1477:u16, "VBIN"=w1482:u16, "HBIN"=w1513:u16, "PREAMP"=w1481:u8, "EM_GAIN"=w1480:u16, "READOUT_RATE"=w1475:u8, "SHUTTER_OPENNING_TIME"=w1512:u16, "SHUTTER_CLOSING_TIME"=w1511:u16, "VERTICAL_SHIFT_SPEED"=w1510:u8, "READ_MODE"=w1509:u8, "VERTICAL_CLOCK_VOLTAGE"=w1508:u8, "AD_CHANNEL"=w1507:u32, "SHUTTER_MODE"=w1504:u8, "SHUTTER_TTL"=w1505:u8, "TRIGGER_MODE"=w1483:u8, "FRAME_TRANSFER"=w1484:bool, "ACQUISITION_MODE"=w1506:u8, "EM_MODE"=w1474:u8)
                n821 = local read "CH2on"() -> (w1464:bool)
                n822 = case shown="False" w1464 {
                  tunnel: w1503 -> [_ w1544]
                  tunnel: w1502 -> [_ w1543]
                  tunnel: w1501 -> [_ w1542]
                  tunnel: w1500 -> [_ w1541]
                  tunnel: w1499 -> [_ w1540]
                  tunnel: w1498 -> [_ w1539]
                  tunnel: w1497 -> [_ w1538]
                  tunnel: w1496 -> [_ w1537]
                  tunnel: w1495 -> [_ w1536]
                  tunnel: w1494 -> [_ w1535]
                  tunnel: w1493 -> [_ w1534]
                  tunnel: w1492 -> [_ w1533]
                  tunnel: w1491 -> [_ w1532]
                  tunnel: w1490 -> [_ w1531]
                  tunnel: w1489 -> [_ w1530]
                  tunnel: w1488 -> [_ w1529]
                  tunnel: w1487 -> [_ w1528]
                  tunnel: w1486 -> [_ w1527]
                  tunnel: w1462 -> [_ w1526]
                  tunnel: w1461 -> [_ w1525]
                  tunnel: w1485 -> [_ w1524]
                  tunnel: [T12."Disabled and Grayed Out" ("Disabled") T12."Enabled" ("Disabled")] -> w1463
                  frame False {
                    w1522 = FALSE ("Blinking")
                    n823 = property on="Image FInal Column 2" class="DigNum (strict)"("Blinking"=w1522) -> ()  [unwired: 2 in, 2 out]
                    n824 = property on="Frame Transfer 2" class="Bool (strict)"("Blinking"=w1522) -> ()  [unwired: 2 in, 2 out]
                    n825 = property on="Vertical Clock Voltage 2" class="Ring (strict)"("Blinking"=w1522) -> ()  [unwired: 2 in, 2 out]
                    n826 = property on="A/D Channel 2" class="DigNum (strict)"("Blinking"=w1522) -> ()  [unwired: 2 in, 2 out]
                    n827 = property on="Image Initial Line 2" class="DigNum (strict)"("Blinking"=w1522) -> ()  [unwired: 2 in, 2 out]
                    n828 = property on="Image Initial Column 2" class="DigNum (strict)"("Blinking"=w1522) -> ()  [unwired: 2 in, 2 out]
                    n829 = property on="Image Final Line 2" class="DigNum (strict)"("Blinking"=w1522) -> ()  [unwired: 2 in, 2 out]
                    n830 = property on="Shutter Openning Time 2" class="DigNum (strict)"("Blinking"=w1522) -> ()  [unwired: 2 in, 2 out]
                    n831 = property on="Shutter Closing Time 2" class="DigNum (strict)"("Blinking"=w1522) -> ()  [unwired: 2 in, 2 out]
                    n832 = property on="Vertical Binning 2" class="DigNum (strict)"("Blinking"=w1522) -> ()  [unwired: 2 in, 2 out]
                    n833 = property on="Horizontal Binning 2" class="DigNum (strict)"("Blinking"=w1522) -> ()  [unwired: 2 in, 2 out]
                    n834 = property on="CCD EM Gain 2" class="DigNum (strict)"("Blinking"=w1522) -> ()  [unwired: 2 in, 2 out]
                    n835 = property on="Shutter Mode 2" class="Ring (strict)"("Blinking"=w1522) -> ()  [unwired: 2 in, 2 out]
                    n836 = property on="Shutter TTL 2" class="Ring (strict)"("Blinking"=w1522) -> ()  [unwired: 2 in, 2 out]
                    n837 = property on="Acquisition Mode 2" class="Ring (strict)"("Blinking"=w1522) -> ()  [unwired: 2 in, 2 out]
                    n838 = property on="Readout Rate 2" class="Ring (strict)"("Blinking"=w1522) -> ()  [unwired: 2 in, 2 out]
                    n839 = property on="Vertical Shift Speed 2" class="Ring (strict)"("Blinking"=w1522) -> ()  [unwired: 2 in, 2 out]
                    n840 = property on="CCD EM Mode 2" class="Ring (strict)"("Blinking"=w1522) -> ()  [unwired: 2 in, 2 out]
                    n841 = property on="Trigger Mode 2" class="Ring (strict)"("Blinking"=w1522) -> ()  [unwired: 2 in, 2 out]
                    n842 = property on="Read Mode 2" class="Ring (strict)"("Blinking"=w1522) -> ()  [unwired: 2 in, 2 out]
                    n843 = property on="Pre-amplification Gain 2" class="Ring (strict)"("Blinking"=w1522) -> ()  [unwired: 2 in, 2 out]
                  }
                  frame True {
                    n844 = Not(x=w1541) -> (.not. x?=w1562:bool)
                    n845 = Not(x=w1540) -> (.not. x?=w1560:bool)
                    n846 = Not(x=w1539) -> (.not. x?=w1561:bool)
                    n847 = Not(x=w1538) -> (.not. x?=w1559:bool)
                    n848 = Not(x=w1544) -> (.not. x?=w1564:bool)
                    n849 = Not(x=w1543) -> (.not. x?=w1563:bool)
                    n850 = Not(x=w1542) -> (.not. x?=w1565:bool)
                    n851 = property on="Image FInal Column 2" class="DigNum (strict)"("Blinking"=w1562) -> ()  [unwired: 2 in, 2 out]
                    n852 = property on="Frame Transfer 2" class="Bool (strict)"("Blinking"=w1560) -> ()  [unwired: 2 in, 2 out]
                    n853 = property on="Vertical Clock Voltage 2" class="Ring (strict)"("Blinking"=w1561) -> ()  [unwired: 2 in, 2 out]
                    n854 = property on="A/D Channel 2" class="DigNum (strict)"("Blinking"=w1559) -> ()  [unwired: 2 in, 2 out]
                    n855 = property on="Image Initial Line 2" class="DigNum (strict)"("Blinking"=w1564) -> ()  [unwired: 2 in, 2 out]
                    n856 = property on="Image Initial Column 2" class="DigNum (strict)"("Blinking"=w1563) -> ()  [unwired: 2 in, 2 out]
                    n857 = property on="Image Final Line 2" class="DigNum (strict)"("Blinking"=w1565) -> ()  [unwired: 2 in, 2 out]
                    n858 = Not(x=w1534) -> (.not. x?=w1555:bool)
                    n859 = Not(x=w1533) -> (.not. x?=w1557:bool)
                    n860 = Not(x=w1532) -> (.not. x?=w1556:bool)
                    n861 = Not(x=w1531) -> (.not. x?=w1558:bool)
                    n862 = Not(x=w1537) -> (.not. x?=w1553:bool)
                    n863 = Not(x=w1536) -> (.not. x?=w1554:bool)
                    n864 = Not(x=w1535) -> (.not. x?=w1552:bool)
                    n865 = property on="Shutter Openning Time 2" class="DigNum (strict)"("Blinking"=w1555) -> ()  [unwired: 2 in, 2 out]
                    n866 = property on="Shutter Closing Time 2" class="DigNum (strict)"("Blinking"=w1557) -> ()  [unwired: 2 in, 2 out]
                    n867 = property on="Vertical Binning 2" class="DigNum (strict)"("Blinking"=w1556) -> ()  [unwired: 2 in, 2 out]
                    n868 = property on="Horizontal Binning 2" class="DigNum (strict)"("Blinking"=w1558) -> ()  [unwired: 2 in, 2 out]
                    n869 = property on="CCD EM Gain 2" class="DigNum (strict)"("Blinking"=w1553) -> ()  [unwired: 2 in, 2 out]
                    n870 = property on="Shutter Mode 2" class="Ring (strict)"("Blinking"=w1554) -> ()  [unwired: 2 in, 2 out]
                    n871 = property on="Shutter TTL 2" class="Ring (strict)"("Blinking"=w1552) -> ()  [unwired: 2 in, 2 out]
                    n872 = Not(x=w1530) -> (.not. x?=w1545:bool)
                    n873 = Not(x=w1526) -> (.not. x?=w1548:bool)
                    n874 = Not(x=w1525) -> (.not. x?=w1546:bool)
                    n875 = Not(x=w1524) -> (.not. x?=w1547:bool)
                    n876 = Not(x=w1529) -> (.not. x?=w1550:bool)
                    n877 = Not(x=w1528) -> (.not. x?=w1549:bool)
                    n878 = Not(x=w1527) -> (.not. x?=w1551:bool)
                    n879 = property on="Acquisition Mode 2" class="Ring (strict)"("Blinking"=w1545) -> ()  [unwired: 2 in, 2 out]
                    n880 = property on="Readout Rate 2" class="Ring (strict)"("Blinking"=w1548) -> ()  [unwired: 2 in, 2 out]
                    n881 = property on="Vertical Shift Speed 2" class="Ring (strict)"("Blinking"=w1546) -> ()  [unwired: 2 in, 2 out]
                    n882 = property on="CCD EM Mode 2" class="Ring (strict)"("Blinking"=w1547) -> ()  [unwired: 2 in, 2 out]
                    n883 = property on="Trigger Mode 2" class="Ring (strict)"("Blinking"=w1550) -> ()  [unwired: 2 in, 2 out]
